vi "Update Lift Position.vi"(0 "Top Limit":bool, 5 "Upper Limit":bool, 7 "Middle Limit":bool, 9 "Lower Limit":bool, 11 "Bottom Limit":bool) -> ()   [LabVIEW 2014]
uses:
  Robot Global Data.vi
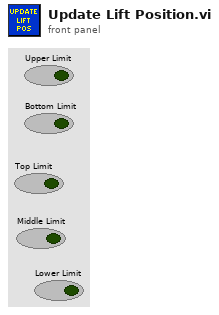
[diagram p1: front panel]
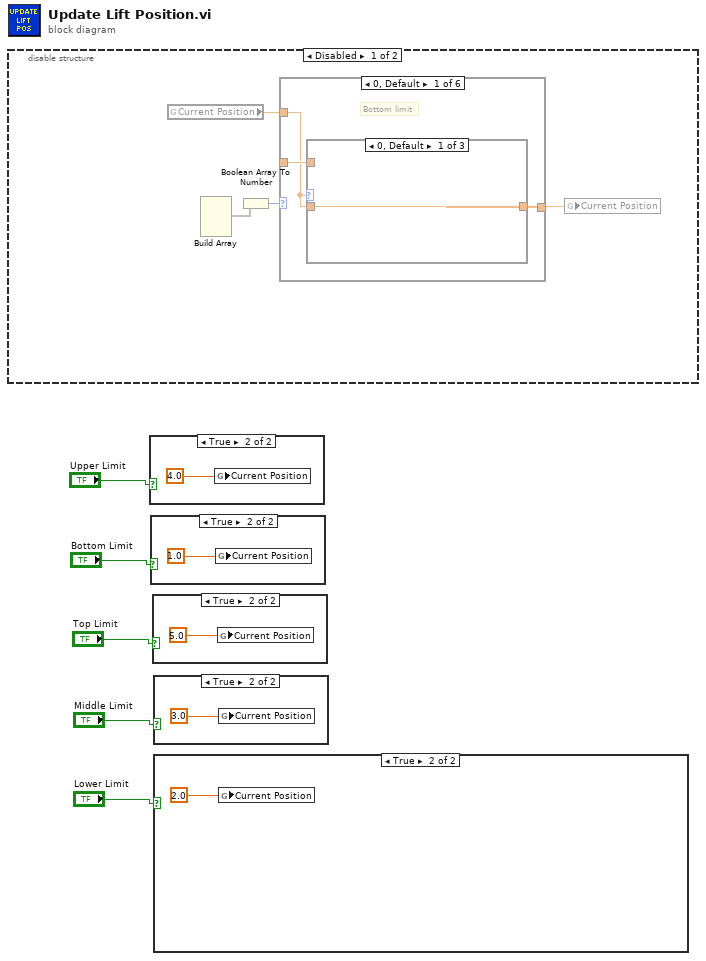
[diagram p0: block diagram]
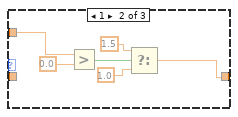
[diagram p2: hidden frame]
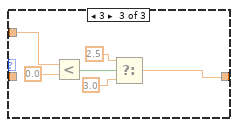
[diagram p3: hidden frame]
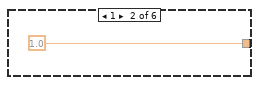
[diagram p4: hidden frame]
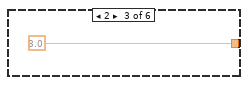
[diagram p5: hidden frame]
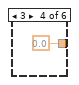
[diagram p6: hidden frame]
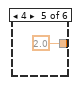
[diagram p7: hidden frame]
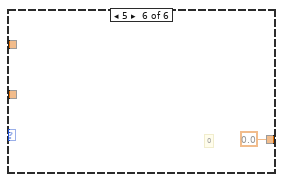
[diagram p8: hidden frame]
diagram:
  n1 = disable-structure shown="Disabled" {
    frame Disabled {
      n2 = global read "Robot Global Data.vi" "Current Position"() -> (w10:dbl)
      n3 = Build Array() -> (w15:void[], w13:dbl, w12:dbl, w9:dbl, w7:dbl, w8:dbl)
      n4 = Boolean Array To Number(Boolean array=w15) -> (number=w6:u32)
      n5 = case shown="0, Default" w6 {
        tunnel: [w18 1.0 ("Current Position") 3.0 ("Current Position") 0.0 ("Current Position") 2.0 ("Current Position") 0.0 ("Current Position")] -> w14
        tunnel: [w17 _ _ _ _ _] -> w11
        tunnel: w10 -> [w16 _ _ _ _ _]
        frame 0, Default {
          # "Bottom limit"
          n6 = case shown="0, Default" w16 {
            tunnel: [w19 w20 w27] -> w18
            tunnel: w17 -> [_ w25 w26]
            tunnel: w16 -> [w19 _ _]
            frame 0, Default {
            }
            frame 1 {
              n7 = Greater?(x=w25, y=0.0) -> (0:w23:bool)
              n8 = Select(t=1.5, s=w23, f=1.0) -> (s? t:f=w20:dbl)
            }
            frame 3 {
              n9 = Less?(x=w26, y=0.0) -> (x < y?=w30:bool)
              n10 = Select(t=2.5, s=w30, f=3.0) -> (s? t:f=w27:dbl)
            }
          }
        }
        frame 1 {
        }
        frame 2 {
        }
        frame 3 {
        }
        frame 4 {
        }
        frame 5 {
          # "0"
        }
      }
      n11 = global write "Robot Global Data.vi" "Current Position"(w14) -> ()
    }
    frame Enabled {
    }
  }
  n12 = case shown="True" "Upper Limit" {
    frame False {
    }
    frame True {
      n13 = global write "Robot Global Data.vi" "Current Position"(4.0) -> ()
    }
  }
  n14 = case shown="True" "Bottom Limit" {
    frame False {
    }
    frame True {
      n15 = global write "Robot Global Data.vi" "Current Position"(1.0) -> ()
    }
  }
  n16 = case shown="True" "Top Limit" {
    frame False {
    }
    frame True {
      n17 = global write "Robot Global Data.vi" "Current Position"(5.0) -> ()
    }
  }
  n18 = case shown="True" "Middle Limit" {
    frame False {
    }
    frame True {
      n19 = global write "Robot Global Data.vi" "Current Position"(3.0) -> ()
    }
  }
  n20 = case shown="True" "Lower Limit" {
    frame False {
    }
    frame True {
      n21 = global write "Robot Global Data.vi" "Current Position"(2.0) -> ()
    }
  }
